vi "SSL Detection Balls Invalidate.vi"(11 "Value":T1[](array[typedef])) -> (3 "Array":T1[](array[typedef]))   [LabVIEW 2016]
uses:
  SSL Detection Ball.ctl
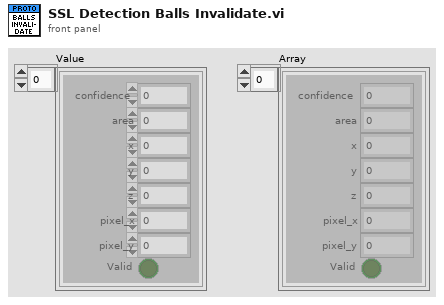
[diagram p1: front panel]
types:
  T1 = typedef "SSL Detection Ball.ctl" = cluster{"x":sgl, "area":u32, "confidence":sgl, "y":sgl, "z":sgl, "pixel_x":sgl, "pixel_y":sgl, "Valid":bool}
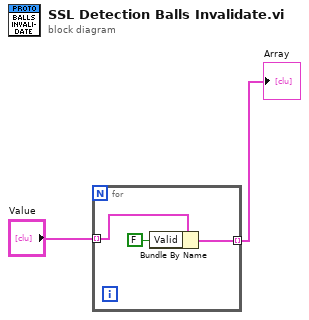
[diagram p0: block diagram]
diagram:
  n1 = for {
    tunnel: "Value" -> [w5] mode=indexing
    tunnel: [w3] -> w2 mode=indexing
    n2 = Bundle By Name(cluster=w5, "Valid"=FALSE) -> (w3:T1)
  }
  "Array" <- w2
